vi "GlobePSUVoltagesStore.vi"(8 "error in (no error)":errorcluster, 10 "Experiment State":T1 {"Global Settings"."Initial Background Values"."Cryo temp [K]" format="%#_4g"; "RIO Settings"."Card Settings"."Sample Rate" format="%#_3p"; "Timing Settings"."Timing Channel Settings"."FrontPanelTime" format="%.3p"; "Timing Settings"."Timing Channel Settings"."Pulse width (s)" format="%.3p"; "Timing Settings"."Timing Channel Settings"."Delay (s)" format="%.3p"; "DAQ Settings"."Card Settings"."Global Edge Type" items=["Rising"=10280, "Falling"=10171]; "DAQ Settings"."Card Settings"."Sample Rate" format="%#_3p"}, 11 "Tree DVR in":refnum<data-value>) -> (0 "error out":errorcluster)   [LabVIEW 2014]
uses:
  <vilib>/MDSplus/Classes/Tree_Class/Tree.lvclass
  Controls/ExperimentStateCluster.ctl
  Controls/DigitizerSettingsChannelSettings.ctl
  Controls/DigitizerSettingsCardSettingsArray.ctl
  Controls/DigitizerSettingsCardSettings.ctl
  Controls/TimingSettings.ctl
  Controls/TimingCardSettings.ctl
  Controls/TimingChannelSettings.ctl
  Controls/RIOSettingsExperimentStateCluster.ctl
  Controls/RIOChannelSettingsArrayExperimentStateCluster.ctl
  Controls/RIOSettingsChannelSettings.ctl
  Controls/RIOSettingsCardSettingsArray.ctl
  Controls/RIOSettingsCardSettings.ctl
  <vilib>/userdefined/High Color/nirio_resource_hc.ctl
  Controls/RIOData.ctl
  Controls/DIOChannel.ctl
  Controls/TachometerControls.ctl
  Controls/Global Settings/GlobalSettings.ctl
  Controls/Global Settings/InitialBackgroundValues.ctl
  Controls/Global Settings/GasPuffing.ctl
  Controls/Global Settings/PSUVoltages.ctl
  Controls/Global Settings/ScopeDetails.ctl
  Controls/Calibrations/Calibrations.ctl
  Controls/Calibrations/CryoTemoCalibration.ctl
  Controls/Calibrations/PSU2TachCalibration.ctl
  Controls/Calibrations/PSU3TachCalibration.ctl
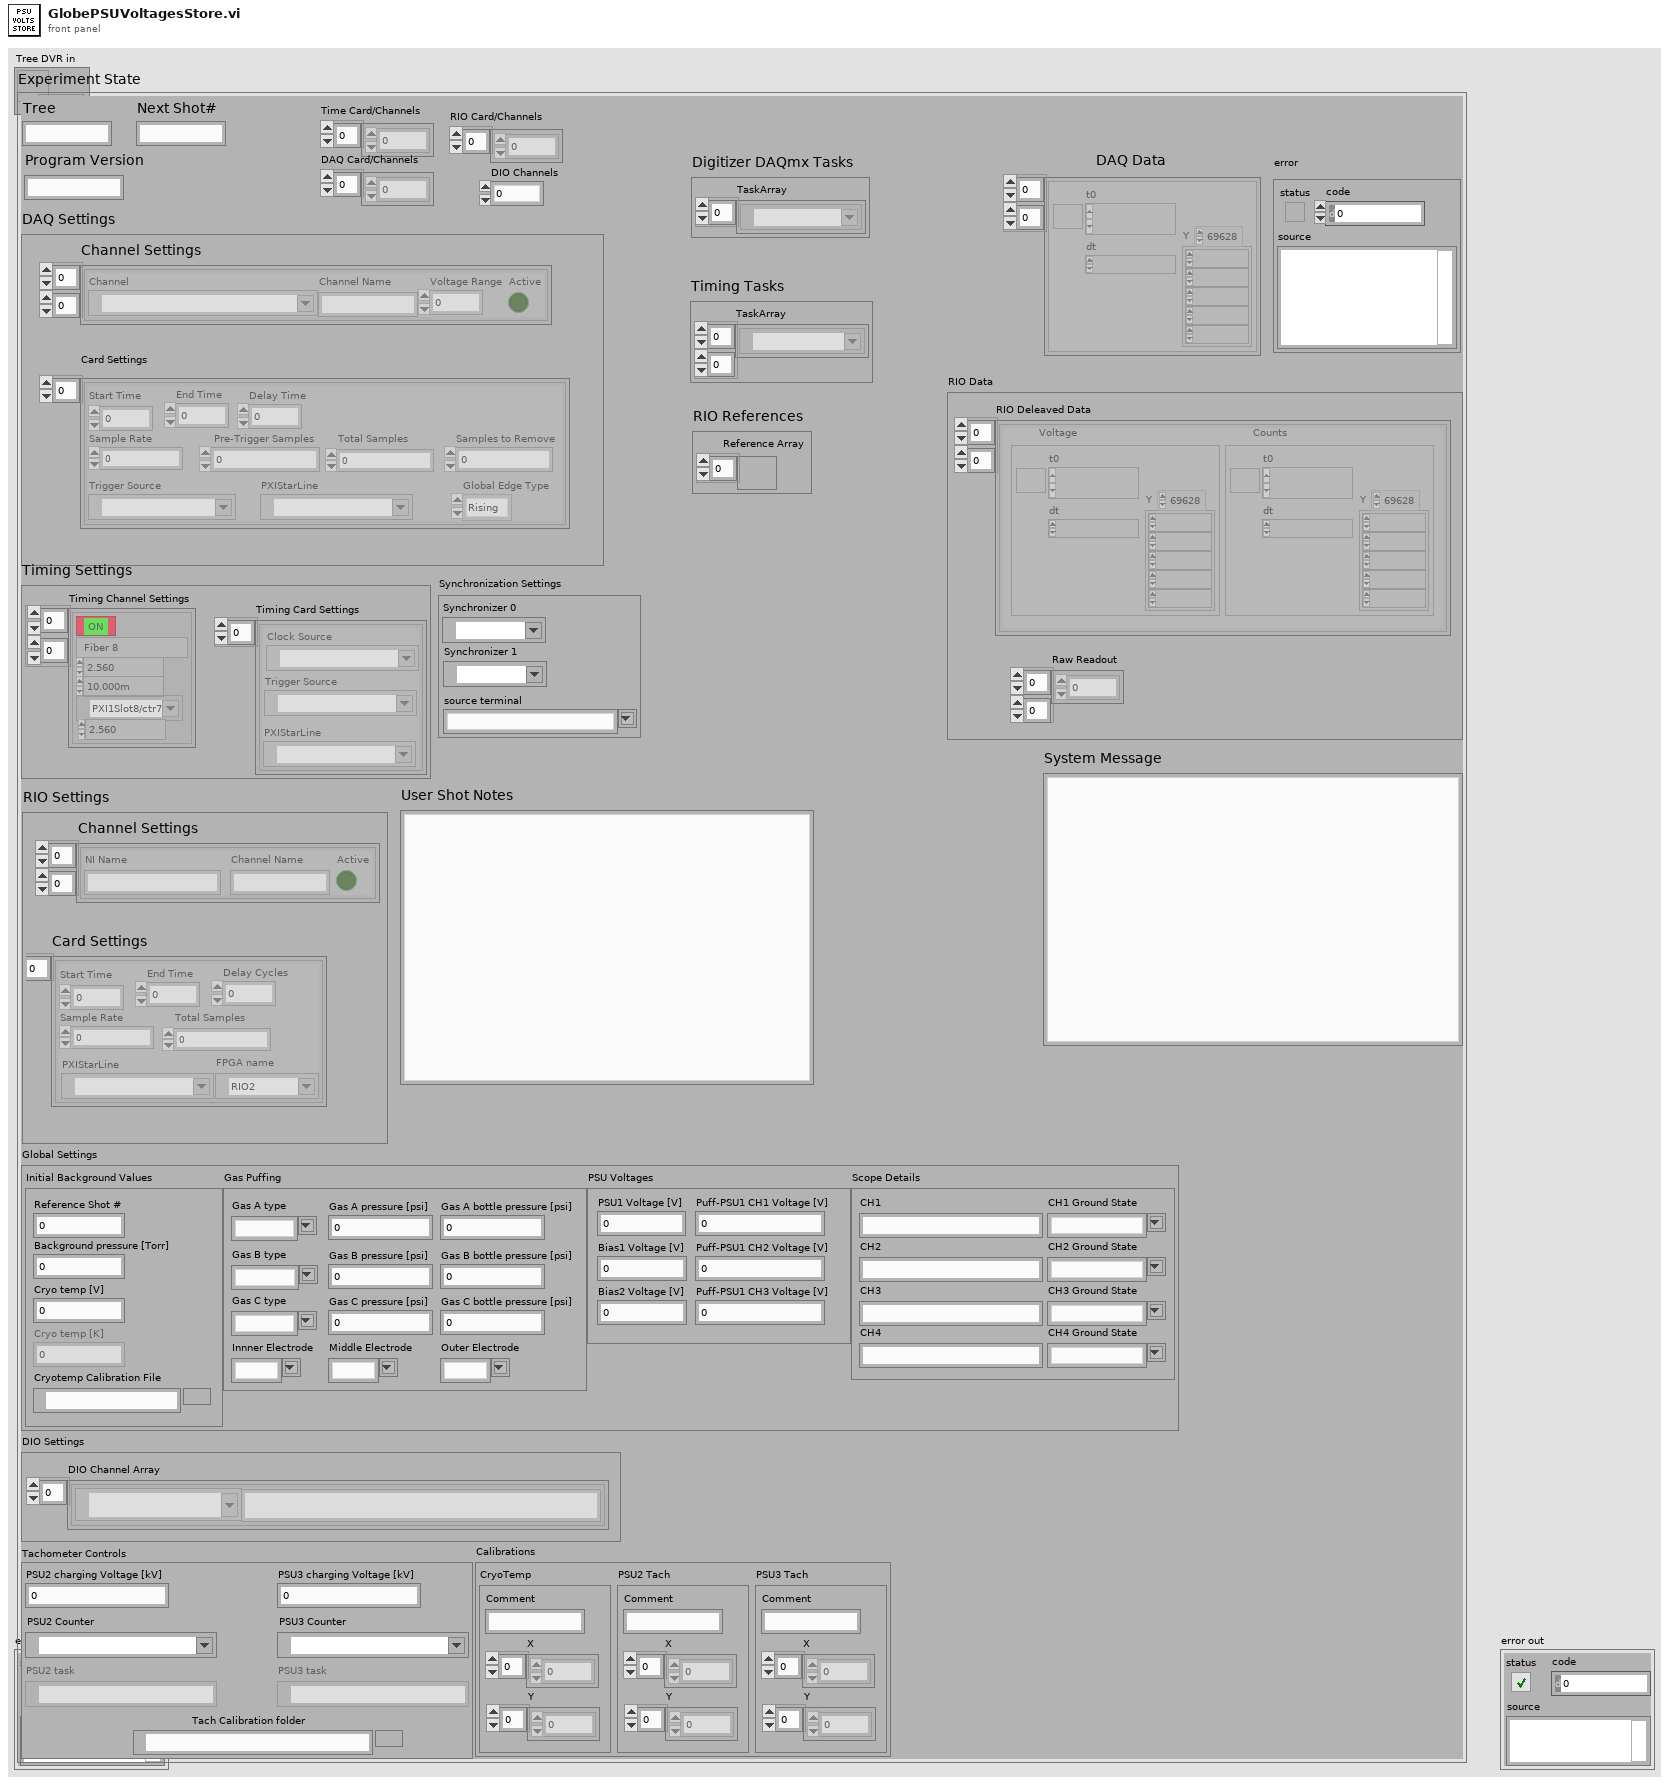
[diagram p1: front panel]
types:
  T1 = typedef "ExperimentStateCluster.ctl" = cluster{"error":errorcluster, "Digitizer DAQmx Tasks":cluster{"TaskArray":refnum<k21>[]}, "DAQ Settings":cluster{"Channel Settings":T2[][], "Card Settings":T3}, "Synchronization Settings":cluster{"Synchronizer 0":refnum<k15>, "source terminal":string, "Synchronizer 1":refnum<k15>}, "DAQ Data":waveform(dbl)[][], "Next Shot#":string, "System Message":string, "User Shot Notes":string, "Timing Settings":T5, "Timing Tasks":cluster{"TaskArray":refnum<k21>[][]}, "Tree":string, "Time Card/Channels":i32[], "DAQ Card/Channels":i32[], "Program Version":string, "RIO Settings":T8, "RIO References":cluster{"Reference Array":refnum<k20>[]}, "RIO Data":T14, "RIO Card/Channels":i32[], "DIO Channels":i32, "DIO Settings":cluster{"DIO Channel Array":T15[]}, "Tachometer Controls":T16, "Global Settings":T17, "Calibrations":T22}
  T2 = typedef "DigitizerSettingsChannelSettings.ctl" = cluster{"Channel":tag, "Channel Name":string, "Voltage Range":dbl, "Active":bool}
  T3 = typedef "DigitizerSettingsCardSettingsArray.ctl" = T4[]
  T4 = typedef "DigitizerSettingsCardSettings.ctl" = cluster{"Start Time":dbl, "End Time":dbl, "Sample Rate":dbl, " Pre-Trigger Samples":u32, "Total Samples":i32, "Samples to Remove":u32, "Trigger Source":tag, "Global Edge Type":i32, "PXIStarLine":tag, "Delay Time":dbl}
  T5 = typedef "TimingSettings.ctl" = cluster{"Timing Card Settings":T6[], "Timing Channel Settings":T7[][]}
  T6 = typedef "TimingCardSettings.ctl" = cluster{"Trigger Source":tag, "Clock Source":tag, "PXIStarLine":tag}
  T7 = typedef "TimingChannelSettings.ctl" = cluster{"Delay (s)":dbl, "Pulse width (s)":dbl, "Active":bool, "Channel Name":string, "counter":tag, "FrontPanelTime":dbl}
  T8 = typedef "RIOSettingsExperimentStateCluster.ctl" = cluster{"Channel Settings":T9, "Card Settings":T11}
  T9 = typedef "RIOChannelSettingsArrayExperimentStateCluster.ctl" = T10[][]
  T10 = typedef "RIOSettingsChannelSettings.ctl" = cluster{"Channel Name":string, "Active":bool, "NI Name":string}
  T11 = typedef "RIOSettingsCardSettingsArray.ctl" = T12[]
  T12 = typedef "RIOSettingsCardSettings.ctl" = cluster{"Start Time":dbl, "End Time":dbl, "Sample Rate":dbl, "Total Samples":u64, "PXIStarLine":tag, "Delay Cycles":u64, "FPGA name":T13}
  T13 = typedef "nirio_resource_hc.ctl" = tag
  T14 = typedef "RIOData.ctl" = cluster{"RIO Deleaved Data":cluster{"Voltage":waveform(dbl), "Counts":waveform(i16)}[][], "Raw Readout":u64[][]}
  T15 = typedef "DIOChannel.ctl" = cluster{"Channel Name":string, "NI Name":tag}
  T16 = typedef "TachometerControls.ctl" = cluster{"Tach Calibration folder":path, "PSU2 charging Voltage [kV]":dbl, "PSU2 Counter":tag, "PSU2 task":refnum<k21>, "PSU3 Counter":tag, "PSU3 task":refnum<k21>, "PSU3 charging Voltage [kV]":dbl}
  T17 = typedef "GlobalSettings.ctl" = cluster{"Initial Background Values":T18, "Gas Puffing":T19, "PSU Voltages":T20, "Scope Details":T21}
  T18 = typedef "InitialBackgroundValues.ctl" = cluster{"Reference Shot #":dbl, "Background pressure [Torr]":dbl, "Cryo temp [V]":dbl, "Cryo temp [K]":dbl, "Cryotemp Calibration File":path}
  T19 = typedef "GasPuffing.ctl" = cluster{"Gas A type":string, "Gas B type":string, "Gas C type":string, "Gas A pressure [psi]":dbl, "Gas B pressure [psi]":dbl, "Gas C pressure [psi]":dbl, "Innner Electrode":string, "Middle Electrode":string, "Outer Electrode":string, "Gas A bottle pressure [psi]":dbl, "Gas B bottle pressure [psi]":dbl, "Gas C bottle pressure [psi]":dbl}
  T20 = typedef "PSUVoltages.ctl" = cluster{"Bias1 Voltage [V]":dbl, "Bias2 Voltage [V]":dbl, "PSU1 Voltage [V]":dbl, "Puff-PSU1 CH1 Voltage [V]":dbl, "Puff-PSU1 CH2 Voltage [V]":dbl, "Puff-PSU1 CH3 Voltage [V]":dbl}
  T21 = typedef "ScopeDetails.ctl" = cluster{"CH1":string, "CH2":string, "CH3":string, "CH4":string, "CH1 Ground State":string, "CH2 Ground State":string, "CH3 Ground State":string, "CH4 Ground State":string}
  T22 = typedef "Calibrations.ctl" = cluster{"CryoTemp":T23, "PSU2 Tach":T24, "PSU3 Tach":T25}
  T23 = typedef "CryoTemoCalibration.ctl" = cluster{"Comment":string, "X":dbl[], "Y":dbl[]}
  T24 = typedef "PSU2TachCalibration.ctl" = cluster{"Comment":string, "X":dbl[], "Y":dbl[]}
  T25 = typedef "PSU3TachCalibration.ctl" = cluster{"Comment":string, "X":dbl[], "Y":dbl[]}
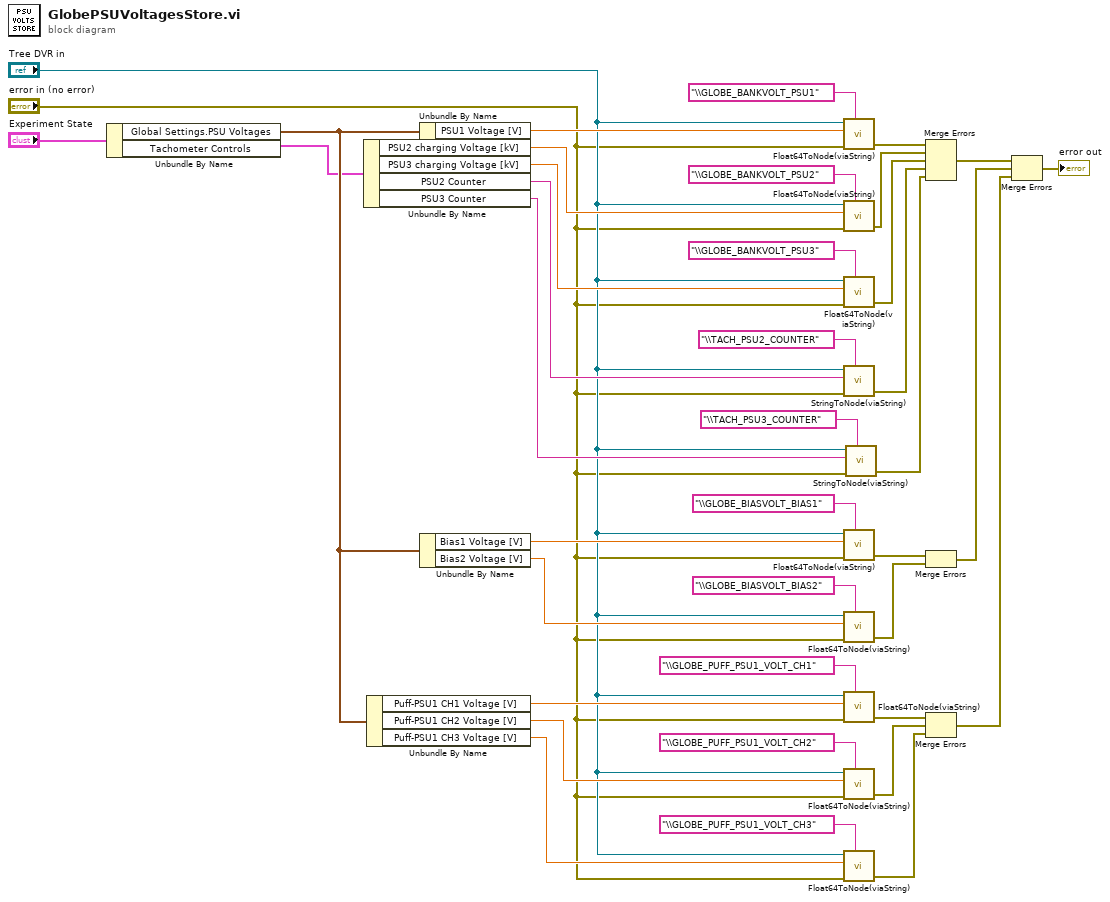
[diagram p0: block diagram]
diagram:
  n1 = Unbundle By Name("Experiment State") -> ("Global Settings.PSU Voltages"=w11:T20, "Tachometer Controls"=w10:T16)
  n2 = Unbundle By Name(w10) -> ("PSU2 charging Voltage [kV]"=w33:dbl, "PSU3 charging Voltage [kV]"=w34:dbl, "PSU2 Counter"=w7:tag, "PSU3 Counter"=w5:tag)
  n3 = Unbundle By Name(w11) -> ("Puff-PSU1 CH1 Voltage [V]"=w37:dbl, "Puff-PSU1 CH2 Voltage [V]"=w38:dbl, "Puff-PSU1 CH3 Voltage [V]"=w39:dbl)
  n4 = Unbundle By Name(w11) -> ("PSU1 Voltage [V]"=w32:dbl)
  n5 = Unbundle By Name(w11) -> ("Bias1 Voltage [V]"=w35:dbl, "Bias2 Voltage [V]"=w36:dbl)
  n6 = call "Float64ToNode(viaString).vi"("Tree DVR in"="Tree DVR in", "DBL in"=w32, "error in"="error in (no error)", "NodePath"="\\GLOBE_BANKVOLT_PSU1") -> ("error out"=w24:errorcluster)  [unwired: 3 in]
  n7 = call "Float64ToNode(viaString).vi"("Tree DVR in"="Tree DVR in", "DBL in"=w33, "error in"="error in (no error)", "NodePath"="\\GLOBE_BANKVOLT_PSU2") -> ("error out"=w25:errorcluster)  [unwired: 3 in]
  n8 = call "Float64ToNode(viaString).vi"("Tree DVR in"="Tree DVR in", "DBL in"=w34, "error in"="error in (no error)", "NodePath"="\\GLOBE_BANKVOLT_PSU3") -> ("error out"=w26:errorcluster)  [unwired: 3 in]
  n9 = call "StringToNode(viaString).vi"("Tree DVR in"="Tree DVR in", "String value in"=w7, "error in (no error)"="error in (no error)", "NodePath"="\\TACH_PSU2_COUNTER") -> ("error out"=w4:errorcluster)  [unwired: 3 in]
  n10 = call "Float64ToNode(viaString).vi"("Tree DVR in"="Tree DVR in", "DBL in"=w35, "error in"="error in (no error)", "NodePath"="\\GLOBE_BIASVOLT_BIAS1") -> ("error out"=w27:errorcluster)  [unwired: 3 in]
  n11 = call "Float64ToNode(viaString).vi"("Tree DVR in"="Tree DVR in", "DBL in"=w36, "error in"="error in (no error)", "NodePath"="\\GLOBE_BIASVOLT_BIAS2") -> ("error out"=w28:errorcluster)  [unwired: 3 in]
  n12 = call "Float64ToNode(viaString).vi"("Tree DVR in"="Tree DVR in", "DBL in"=w37, "error in"="error in (no error)", "NodePath"="\\GLOBE_PUFF_PSU1_VOLT_CH1") -> ("error out"=w29:errorcluster)  [unwired: 3 in]
  n13 = call "Float64ToNode(viaString).vi"("Tree DVR in"="Tree DVR in", "DBL in"=w38, "error in"="error in (no error)", "NodePath"="\\GLOBE_PUFF_PSU1_VOLT_CH2") -> ("error out"=w30:errorcluster)  [unwired: 3 in]
  n14 = call "Float64ToNode(viaString).vi"("Tree DVR in"="Tree DVR in", "DBL in"=w39, "error in"="error in (no error)", "NodePath"="\\GLOBE_PUFF_PSU1_VOLT_CH3") -> ("error out"=w31:errorcluster)  [unwired: 3 in]
  n15 = call "StringToNode(viaString).vi"("Tree DVR in"="Tree DVR in", "String value in"=w5, "error in (no error)"="error in (no error)", "NodePath"="\\TACH_PSU3_COUNTER") -> ("error out"=w3:errorcluster)  [unwired: 3 in]
  n16 = Merge Errors(w24, w25, w26, w4, w3) -> (w12:errorcluster)
  n17 = Merge Errors(w27, w28) -> (w13:errorcluster)
  n18 = Merge Errors(w29, w30, w31) -> (w14:errorcluster)
  n19 = Merge Errors(w12, w13, w14) -> (→"error out":errorcluster)
